vi "FilterComplex.vi"(4 "Scan Data In":cdb[][](array[numeric]), 5 "Samp Rate (MHz)":i16, 6 "Filter Prams":T1={"low cutoff"=5, "order"=81, "high cutoff"=35}) -> (0 "Array":cdb[][](array[numeric]), 2 "Filter Params":T1)   [LabVIEW 2022 SP3]
uses:
  <vilib>/Analysis/2dsp.llb/1D Convolution (CDB).vi
  <vilib>/Analysis/NI_AALPro.lvlib
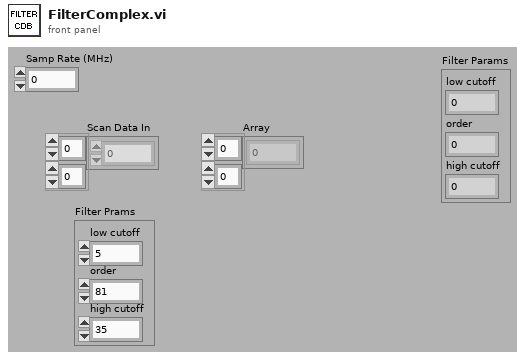
[diagram p1: front panel]
types:
  T1 = cluster{"low cutoff":i32, "order":i32, "high cutoff":i32}
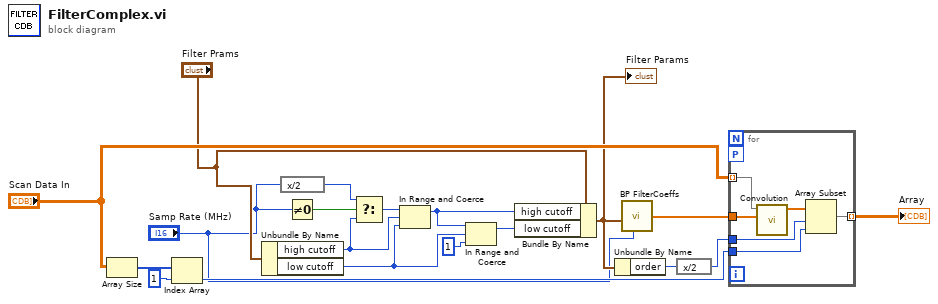
[diagram p0: block diagram]
diagram:
  n1 = Array Size(array="Scan Data In") -> (size(s)=w13:i32[])
  n2 = Index Array(array=w13, index=1) -> (element=w11:i32)
  n3 = Unbundle By Name("Filter Prams") -> ("high cutoff"=w5:i32, "low cutoff"=w3:i32)
  n4 = expression code="x/2"("Samp Rate (MHz)") -> (w7:i16)
  n5 = Not Equal To 0?(x="Samp Rate (MHz)") -> (x != 0?=w8:bool)
  n6 = Select(t=w7, s=w8, f=w5) -> (s? t:f=w6:i32)
  n7 = In Range and Coerce(upper limit=w6, x=w5, lower limit=w3) -> (coerced(x)=w2:i32)  [unwired: 1 out]
  n8 = In Range and Coerce(upper limit=w2, x=w3, lower limit=1) -> (coerced(x)=w1:i32)  [unwired: 1 out]
  n9 = Bundle By Name(cluster="Filter Prams", "high cutoff"=w2, "low cutoff"=w1) -> (w16:T1)
  "Filter Params" <- w16
  n10 = Unbundle By Name(w16) -> ("order"=w15:i32)
  n11 = call "BP FilterCoeffs.vi"("sample rate MHz"="Samp Rate (MHz)", "Filter Prams"=w16) -> ("FIR Windowed Coefficients"=w10:dbl[])  [unwired: 4 in]
  n12 = expression code="x/2"(w15) -> (w14:i32)
  n13 = for {
    tunnel: w14 -> [w21]
    tunnel: [w25] -> w18 mode=indexing
    tunnel: "Scan Data In" -> [w24] mode=indexing
    workers-P: _ -> [_]
    tunnel: w10 -> [w23]
    tunnel: w11 -> [w20]
    n14 = call-poly <vilib>:"Convolution.vi"("Y"=w23, "X"=w24) -> ("X * Y"=w22:cdb[])  [unwired: 1 in, 8 out]
    n15 = Array Subset(array=w22, index=w21, length=w20) -> (w25:cdb[])
  }
  "Array" <- w18
